vi "MakeExample.vi"(8 "error in (no error)":errorcluster, 9 "TriggerRefractoryPeriod (Frames)":i32, 10 "StimulusObject Parameters":variant, 11 "FullWormRailsTriggeredBySmallEllipseRatio in":refnum<class "FullWormRailsTriggeredBySmallEllipseRatio.lvclass">) -> (0 "error out":errorcluster, 3 "FullWormRailsTriggeredBySmallEllipseRatio out":refnum<class "FullWormRailsTriggeredBySmallEllipseRatio.lvclass">)   [LabVIEW 2019, in "FullWormRailsTriggeredBySmallEllipseRatio.lvclass"]
uses:
  FullWormRailsTriggeredBySmallEllipseRatio.lvclass
  FullWormRailsTriggeredBySmallEllipseRatioInputCluster.ctl
  FullWormRailsTriggeredBySmallEllipseRatio.lvclass/FullWormRailsTriggeredBySmallEllipseRatio.ctl
  ParametersGlobal.vi
  StimulusObject.lvclass
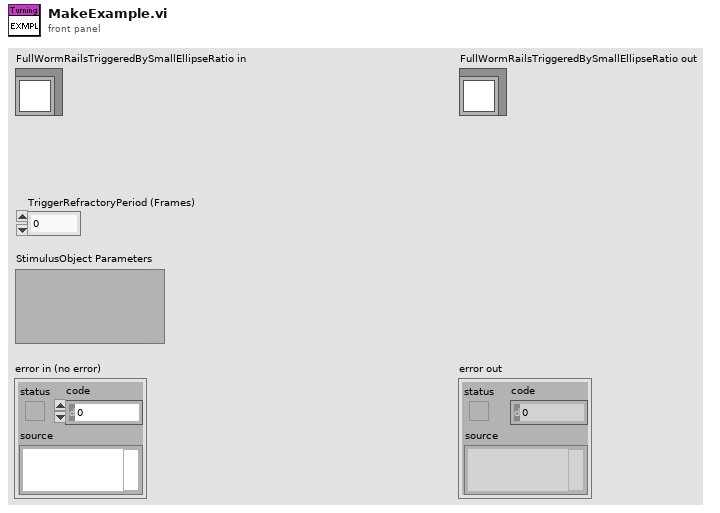
[diagram p1: front panel]
types:
  T1 = typedef "FullWormRailsTriggeredBySmallEllipseRatio.lvclass/FullWormRailsTriggeredBySmallEllipseRatioInputCluster.ctl" = cluster{"Constant Intensity (uW/mm^2, negative is blue)":sgl, "dot radius (mm)":sgl, "Intensities (uW/mm^2, negative is blue)":sgl[], "Durations (s)":sgl[], "Inter trigger interval (s)":dbl, "Ellipse Ratio Trigger Point":sgl, "Turning Preference Parameter":dbl}
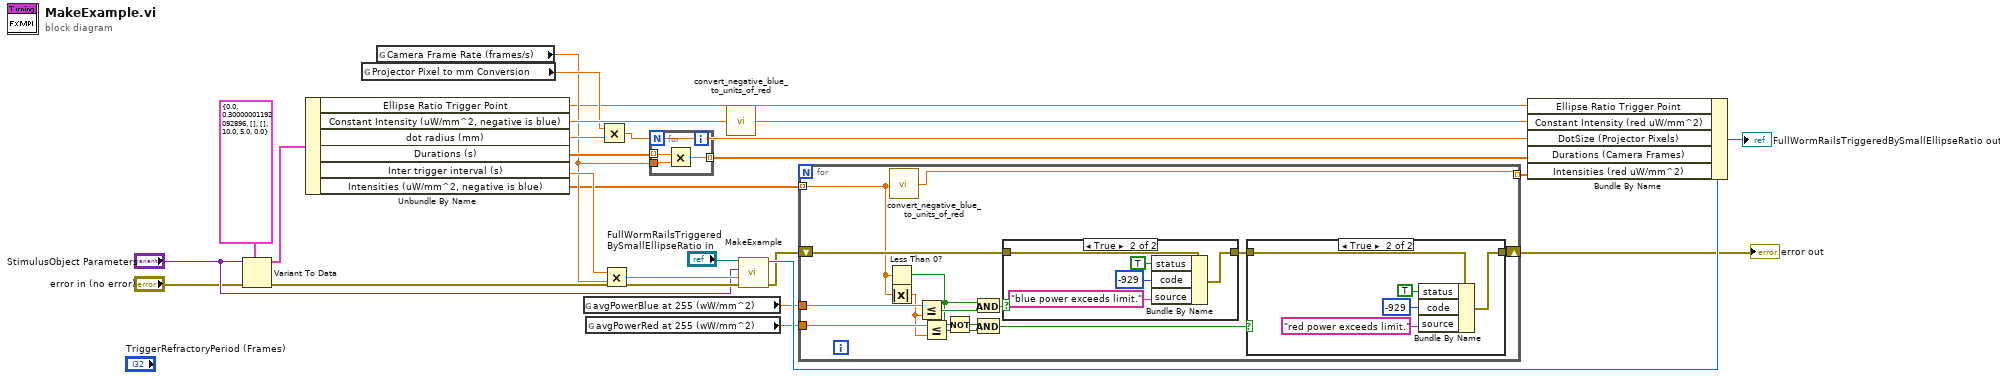
[diagram p0: block diagram]
diagram:
  n1 = Variant To Data(error in="error in (no error)", type=T1 {"Constant Intensity (uW/mm^2, negative is blue)"=0.0, "dot radius (mm)"=0.3, "Intensities (uW/mm^2, negative is blue)"=[], "Durations (s)"=[], "Inter trigger interval (s)"=10.0, "Ellipse Ratio Trigger Point"=5.0, "Turning Preference Parameter"=0.0} ("FullWormRailsInputCluster"), Variant="StimulusObject Parameters") -> (data=w24:T1, error out=w25:errorcluster)
  n2 = Unbundle By Name(w24) -> ("Ellipse Ratio Trigger Point"=w1:sgl, "Constant Intensity (uW/mm^2, negative is blue)"=w20:sgl, "dot radius (mm)"=w18:sgl, "Durations (s)"=w15:sgl[], "Inter trigger interval (s)"=w23:dbl, "Intensities (uW/mm^2, negative is blue)"=w12:sgl[])
  n3 = global read "ParametersGlobal.vi" "Projector Pixel to mm Conversion"() -> (w17:sgl)
  n4 = global read "ParametersGlobal.vi" "Camera Frame Rate (frames/s)"() -> (w14:sgl)
  n5 = global read "ParametersGlobal.vi" "avgPowerBlue at 255 (wW/mm^2)"() -> (w10:sgl)
  n6 = global read "ParametersGlobal.vi" "avgPowerRed at 255 (wW/mm^2)"() -> (w9:sgl)
  n7 = Multiply(x=w17, y=w18) -> (x*y=w16:sgl)
  n8 = Multiply(x=w23, y=w14) -> (x*y=w22:dbl)
  n9 = for {
    tunnel: w15 -> [w28] mode=indexing
    tunnel: w14 -> [w27]
    tunnel: [w26] -> w13 mode=indexing
    n10 = Multiply(x=w28, y=w27) -> (x*y=w26:sgl)
  }
  n11 = call "convert_negative_blue_to_units_of_red.vi"("Intensity in units of red (positive) and blue (negative)"=w20) -> ("Intensity in units of red (positive and negative)"=w19:sgl)
  n12 = call-parent "MakeExample.vi"("error in (no error)"=w25, "TriggerRefractoryPeriod (Frames)"=w22, "StimulusObject Parameters"="StimulusObject Parameters", "StimulusObject in"="FullWormRailsTriggeredBySmallEllipseRatio in") -> ("error out"=w11:errorcluster, "StimulusObject out"=w21:refnum<class "FullWormRailsTriggeredBySmallEllipseRatio.lvclass">)  [unwired: 6 in]
  n13 = for {
    tunnel: w12 -> [w36] mode=indexing
    shift-right: [w40] -> w5
    shift-left: w11 -> [w41]
    tunnel: w10 -> [w39]
    tunnel: w9 -> [w38]
    tunnel: [w37] -> w8 mode=indexing
    n14 = Less Than 0?(x=w36) -> (x < 0?=w29:bool)
    n15 = Absolute Value(x=w36) -> (abs(x)=w35:sgl)
    n16 = call "convert_negative_blue_to_units_of_red.vi"("Intensity in units of red (positive) and blue (negative)"=w36) -> ("Intensity in units of red (positive and negative)"=w37:sgl)
    n17 = Less Or Equal?(x=w39, y=w35) -> (x <= y?=w34:bool)
    n18 = Less Or Equal?(x=w38, y=w35) -> (x <= y?=w31:bool)
    n19 = Not(x=w29) -> (.not. x?=w30:bool)
    n20 = And(x=w29, y=w34) -> (x .and. y?=w33:bool)
    n21 = And(x=w30, y=w31) -> (x .and. y?=w32:bool)
    n22 = case shown="True" w33 {
      tunnel: w41 -> [w49 w54]
      tunnel: [w49 w53] -> w42
      frame False {
      }
      frame True {
        n23 = Bundle By Name(cluster=w54, "status"=TRUE, "code"=-929, "source"="blue power exceeds limit.") -> (w53:errorcluster)
      }
    }
    n24 = case shown="True" w32 {
      tunnel: w42 -> [w43 w48]
      tunnel: [w43 w47] -> w40
      frame False {
      }
      frame True {
        n25 = Bundle By Name(cluster=w48, "status"=TRUE, "code"=-929, "source"="red power exceeds limit.") -> (w47:errorcluster)
      }
    }
  }
  "error out" <- w5
  n26 = Bundle By Name(cluster=w21, "Ellipse Ratio Trigger Point"=w1, "Constant Intensity (red uW/mm^2)"=w19, "DotSize (Projector Pixels)"=w16, "Durations (Camera Frames)"=w13, "Intensities (red uW/mm^2)"=w8) -> (→"FullWormRailsTriggeredBySmallEllipseRatio out":refnum<class "FullWormRailsTriggeredBySmallEllipseRatio.lvclass">)
